vi "reset.vi"(8 "error in (no error)":errorcluster, 11 "PsTti in":refnum<class "PsuTti.lvclass">) -> (0 "error out":errorcluster, 3 "PsTti out":refnum<class "PsuTti.lvclass">)   [LabVIEW 2023, in "PsuTti.lvclass"]
doc: "Reset the instrument to default/factory settings."
uses:
  PsuTti.lvclass
  PsuTti.lvclass/PsuTti.ctl
  driver/Tti-Pl303Qmd.lvlib
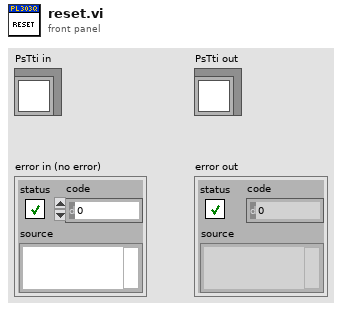
[diagram p1: front panel]
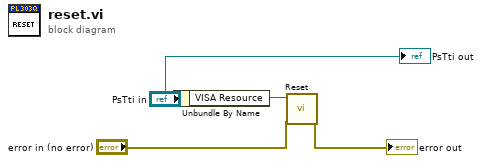
[diagram p0: block diagram]
diagram:
  n1 = Unbundle By Name("PsTti in") -> ("VISA Resource"=w4:refnum<visa-resource-name>)
  n2 = call "Reset.vi"("error in (no error)"="error in (no error)", "VISA resource name"=w4) -> ("error out"=→"error out":errorcluster)  [unwired: 8 in, 1 out]
  "PsTti out" <- "PsTti in"
